vi "AlliGator Convert Gate Image for Export.vi"(8 "error in (no error)":errorcluster, 9 "Exported Gate Image Settings":T1, 10 "Dest Image":T2, 11 "Original Image":T2) -> (0 "error out":errorcluster, 3 "Result Image":T2)   [LabVIEW 2021, in "AlliGator Files.lvlib"]
doc: "Converts a Gate Image (Float) to a U8 or U16 image based on user-selected options."
uses:
  AlliGator Files.lvlib
  <vilib>/vision/Image Controls.llb/IMAQ Image.ctl
  Settings/AlliGator Exported Image Settings.ctl
  <vilib>/Utility/error.llb/Error Cluster From Error Code.vi
  <vilib>/ErrorRing/Error Ring.xnode
  Comparison/Comparison.lvlib
  Settings/AlliGator Settings.lvlib
panel:
  out "dest min value":sgl
  out "dest max value":sgl
  out "source min value":sgl
  out "source max value":sgl
  # "see the AlliGator License on the block diagram (Ctrl+E or Window:Show Block Diagram)"
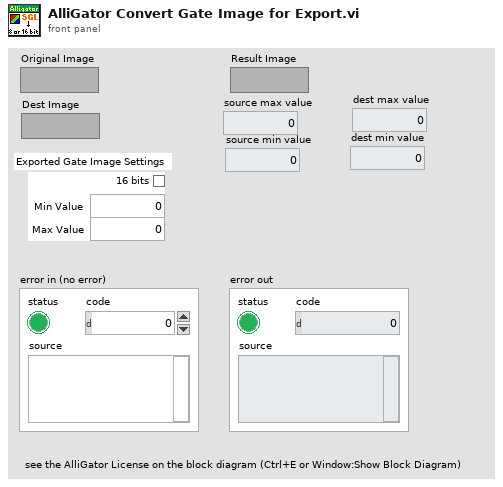
[diagram p1: front panel]
types:
  T1 = typedef "AlliGator Settings.lvlib/AlliGator Exported Image Settings.ctl" = cluster{"bitness":bool, " Min Value":sgl, " Max Value":sgl}
  T2 = typedef "IMAQ Image.ctl" = refnum<image>
  T3 = typedef "Image Type" = u32
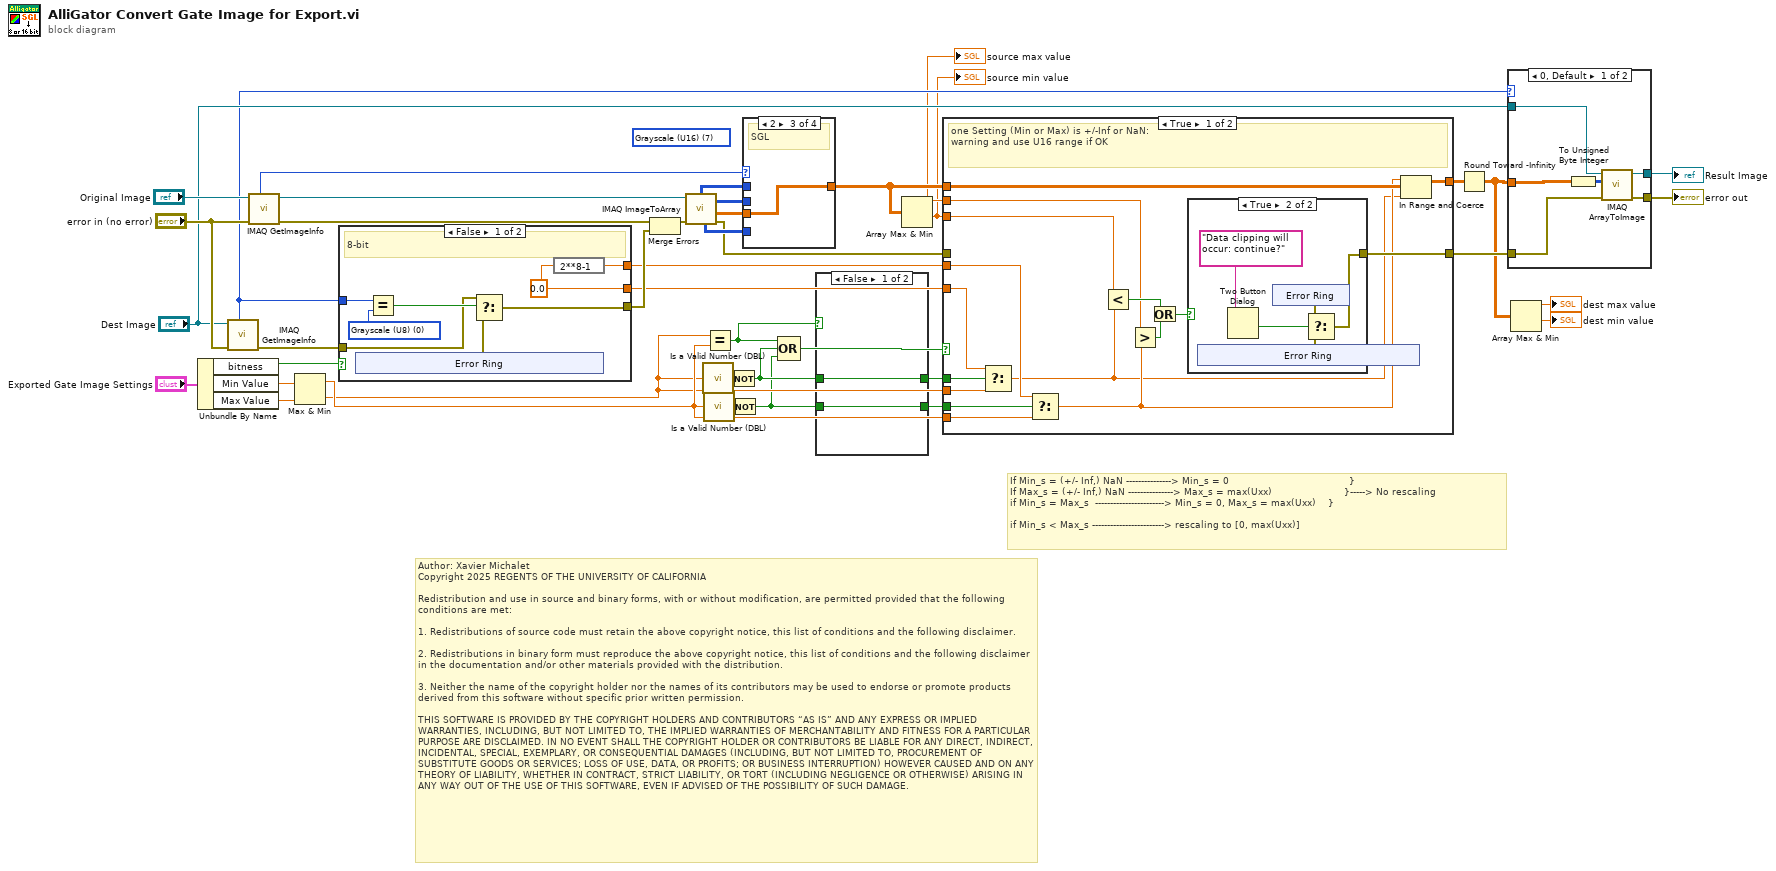
[diagram p0: block diagram]
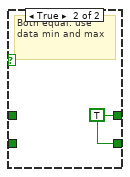
[diagram p2: hidden frame]
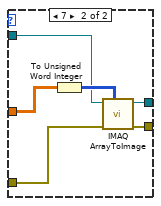
[diagram p3: hidden frame]
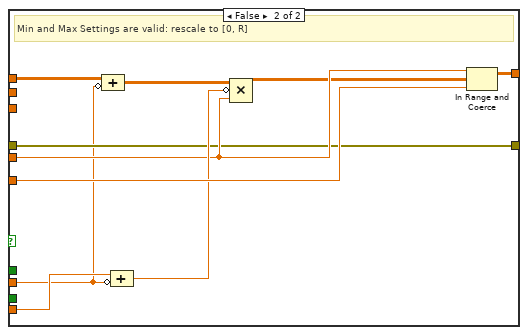
[diagram p5: hidden frame]
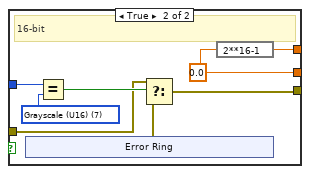
[diagram p6: hidden frame]
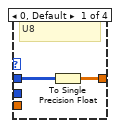
[diagram p7: hidden frame]
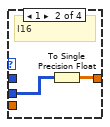
[diagram p8: hidden frame]
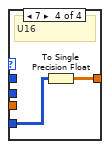
[diagram p9: hidden frame]
diagram:
  (unwired) T3 7 items=["Grayscale (U8)", "Grayscale (I16)", "Grayscale (SGL)", "Complex (CSG)", "RGB (U32)", "HSL (U32)", "RGB (U64)", "Grayscale (U16)"] ("Image Type")
  # "Author: Xavier Michalet\nCopyright 2025 REGENTS OF THE UNIVERSITY OF CALIFORNIA\n\nRedistribution and use in source and binary forms, with or without modification, are permitted provided that the following conditions are met:\n\n1. Redistributions of source code must retain the above copyright notice, this list of conditions and the following disclaimer.\n\n2. Redistributions in binary form must reproduce the above copyright notice, this list of conditions and the following disclaimer in the documentation and/or other materials provided with the distribution.\n\n3. Neither the name of the copyright holder nor the names of its contributors may be used to endorse or promote products derived from this software without specific prior written permission.\n\nTHIS SOFTWARE IS PROVIDED BY THE COPYRIGHT HOLDERS AND CONTRIBUTORS “AS IS” AND ANY EXPRESS OR IMPLIED WARRANTIES, INCLUDING, BUT NOT LIMITED TO, THE IMPLIED WARRANTIES OF MERCHANTABILITY AND FITNESS FOR A PARTICULAR PURPOSE ARE DISCLAIMED. IN NO EVENT SHALL THE COPYRIGHT HOLDER OR CONTRIBUTORS BE LIABLE FOR ANY DIRECT, INDIRECT, INCIDENTAL, SPECIAL, EXEMPLARY, OR CONSEQUENTIAL DAMAGES (INCLUDING, BUT NOT LIMITED TO, PROCUREMENT OF SUBSTITUTE GOODS OR SERVICES; LOSS OF USE, DATA, OR PROFITS; OR BUSINESS INTERRUPTION) HOWEVER CAUSED AND ON ANY THEORY OF LIABILITY, WHETHER IN CONTRACT, STRICT LIABILITY, OR TORT (INCLUDING NEGLIGENCE OR OTHERWISE) ARISING IN ANY WAY OUT OF THE USE OF THIS SOFTWARE, EVEN IF ADVISED OF THE POSSIBILITY OF SUCH DAMAGE."
  # "If Min_s = (+/- Inf,) NaN ---------------> Min_s = 0                                        }\nIf Max_s = (+/- Inf,) NaN ---------------> Max_s = max(Uxx)                        }-----> No rescaling\nif Min_s = Max_s  -----------------------> Min_s = 0, Max_s = max(Uxx)    }\n\nif Min_s < Max_s ------------------------> rescaling to [0, max(Uxx)]"
  n1 = Unbundle By Name("Exported Gate Image Settings") -> ("bitness"=w32:bool, "Min Value"=w9:sgl, "Max Value"=w8:sgl)
  n2 = call "IMAQ GetImageInfo"("error in (no error)"="error in (no error)", "Image"="Dest Image") -> ("error out"=w31:errorcluster, "Image Type"=w19:T3)  [unwired: 2 in, 6 out]
  n3 = call "IMAQ GetImageInfo"("error in (no error)"="error in (no error)", "Image"="Original Image") -> ("error out"=w15:errorcluster, "Image Type"=w39:T3)  [unwired: 2 in, 6 out]
  n4 = Max & Min(x=w9, y=w8) -> (max(x,y)=w5:sgl, min(x,y)=w4:sgl)
  n5 = case shown="False" w32 {
    tunnel: w19 -> [w48 w60]
    tunnel: w31 -> [w45 w57]
    tunnel: [w44 w56] -> w30
    tunnel: [w41 w54] -> w27
    tunnel: [w42 w53] -> w26
    frame False {
      w41 = sgl 0.0 ("Min Value")
      w47 = T3 0 items=["Grayscale (U8)", "Grayscale (I16)", "Grayscale (SGL)", "Complex (CSG)", "RGB (U32)", "HSL (U32)", "RGB (U64)", "Grayscale (U16)"] ("y")
      # "8-bit"
      n6 = xnode "Error Ring"() -> ("error out"=w43:errorcluster)
      n7 = Equal?(x=w48, y=w47) -> (x = y?=w46:bool)
      n8 = Select(t=w45, s=w46, f=w43) -> (s? t:f=w44:errorcluster)
      n9 = expression code="2**8-1"(w41) -> (w42:sgl)
    }
    frame True {
      w54 = sgl 0.0 ("Min Value")
      w59 = T3 7 items=["Grayscale (U8)", "Grayscale (I16)", "Grayscale (SGL)", "Complex (CSG)", "RGB (U32)", "HSL (U32)", "RGB (U64)", "Grayscale (U16)"] ("y")
      # "16-bit"
      n10 = xnode "Error Ring"() -> ("error out"=w55:errorcluster)
      n11 = Equal?(x=w60, y=w59) -> (x = y?=w58:bool)
      n12 = Select(t=w57, s=w58, f=w55) -> (s? t:f=w56:errorcluster)
      n13 = expression code="2**16-1"(w54) -> (w53:sgl)
    }
  }
  n14 = Merge Errors(w15, w30) -> (w16:errorcluster)
  n15 = call "IMAQ ImageToArray"("error in (no error)"=w16, "Image"="Original Image") -> ("Image Pixels (U16)"=w35:u16[][], "Image Pixels (Float)"=w36:sgl[][], "error out"=w18:errorcluster, "Image Pixels (U8)"=w38:u8[][], "Image Pixels (I16)"=w37:i16[][])  [unwired: 2 in]
  n16 = call "Is a Valid Number (DBL).vi"("Number"=w4) -> ("Valid Number?"=w21:bool)  [unwired: 8 in]
  n17 = call "Is a Valid Number (DBL).vi"("Number"=w5) -> ("Valid Number?"=w20:bool)  [unwired: 8 in]
  n18 = Equal?(x=w4, y=w5) -> (x = y?=w7:bool)
  n19 = Not(x=w21) -> (.not. x?=w6:bool)
  n20 = Not(x=w20) -> (.not. x?=w2:bool)
  n21 = case shown="2" w39 {
    tunnel: w38 -> [w66 _ _ _]
    tunnel: w37 -> [_ w68 _ _]
    tunnel: w36 -> [_ _ w69 _]
    tunnel: w35 -> [_ _ _ w71]
    tunnel: [w65 w67 w69 w70] -> w28
    frame 0, Default {
      # "U8"
      n22 = To Single Precision Float(number=w66) -> (single precision float=w65:sgl[][])
    }
    frame 1 {
      # "I16"
      n23 = To Single Precision Float(number=w68) -> (single precision float=w67:sgl[][])
    }
    frame 2 {
      # "SGL"
    }
    frame 7 {
      # "U16"
      n24 = To Single Precision Float(number=w71) -> (single precision float=w70:sgl[][])
    }
  }
  n25 = Compound Arithmetic op=OR(w7, w6, w2) -> (w29:bool)
  n26 = case shown="False" w7 {
    tunnel: w6 -> [w73 _]
    tunnel: [w73 w74] -> w3
    tunnel: w2 -> [w72 _]
    tunnel: [w72 w74] -> w1
    frame False {
    }
    frame True {
      w74 = TRUE
      # "Both equal: use data min and max"
    }
  }
  n27 = Array Max & Min(array=w28) -> (max value=w14:sgl, min value=w13:sgl)  [unwired: 2 out]
  "source max value" <- w14
  "source min value" <- w13
  n28 = case shown="True" w29 {
    tunnel: w28 -> [w87 w110]
    tunnel: w27 -> [w82 w107]
    tunnel: w26 -> [w81 w105]
    tunnel: [w90 w109] -> w25
    tunnel: w5 -> [w80 w102]
    tunnel: w3 -> [w89 _]
    tunnel: w1 -> [w88 _]
    tunnel: w18 -> [_ w104]
    tunnel: [w83 w104] -> w17
    tunnel: w14 -> [w79 _]
    tunnel: w13 -> [w78 _]
    tunnel: w4 -> [w77 w101]
    frame True {
      # "one Setting (Min or Max) is +/-Inf or NaN:\nwarning and use U16 range if OK"
      n29 = Select(t=w82, s=w89, f=w77) -> (s? t:f=w75:sgl)
      n30 = Select(t=w81, s=w88, f=w80) -> (s? t:f=w76:sgl)
      n31 = Less?(x=w78, y=w75) -> (x < y?=w86:bool)
      n32 = Greater?(x=w79, y=w76) -> (0:w85:bool)
      n33 = Or(x=w86, y=w85) -> (x .or. y?=w84:bool)
      n34 = case shown="True" w84 {
        tunnel: [_ w91] -> w83
        frame False {
        }
        frame True {
          n35 = xnode "Error Ring"() -> ("error out"=w92:errorcluster)
          n36 = Two Button Dialog(message="Data clipping will occur: continue?") -> (T button?=w94:bool)  [unwired: 2 in]
          n37 = xnode "Error Ring"() -> ("error out"=w93:errorcluster)
          n38 = Select(t=w93, s=w94, f=w92) -> (s? t:f=w91:errorcluster)
        }
      }
      n39 = In Range and Coerce(upper limit=w76, x=w87, lower limit=w75) -> (coerced(x)=w90:sgl[][])  [unwired: 1 out]
    }
    frame False {
      # "Min and Max Settings are valid: rescale to [0, R]"
      n40 = Compound Arithmetic op=ADD(w110, invert w101) -> (w108:sgl[][])
      n41 = Compound Arithmetic op=ADD(w102, invert w101) -> (w106:sgl)
      n42 = Compound Arithmetic op=MULTIPLY(w108, invert w106, w105) -> (w103:sgl[][])
      n43 = In Range and Coerce(upper limit=w105, x=w103, lower limit=w107) -> (coerced(x)=w109:sgl[][])  [unwired: 1 out]
    }
  }
  n44 = Round Toward -Infinity(1:w25) -> (0:w12:sgl[][])
  n45 = case shown="0, Default" w19 {
    tunnel: [w115 w122] -> w24
    tunnel: [w114 w121] -> w23
    tunnel: w17 -> [w113 w120]
    tunnel: "Dest Image" -> [w112 w118]
    tunnel: w12 -> [w111 w117]
    frame 0, Default {
      n46 = To Unsigned Byte Integer(number=w111) -> (unsigned 8bit integer=w116:u8[][])
      n47 = call "IMAQ ArrayToImage"("error in (no error)"=w113, "Image Pixels (U8)"=w116, "Image"=w112) -> ("error out"=w114:errorcluster, "Image Out"=w115:T2)  [unwired: 7 in]
    }
    frame 7 {
      n48 = To Unsigned Word Integer(number=w117) -> (unsigned 16bit integer=w119:u16[][])
      n49 = call "IMAQ ArrayToImage"("Image Pixels (U16)"=w119, "error in (no error)"=w120, "Image"=w118) -> ("error out"=w121:errorcluster, "Image Out"=w122:T2)  [unwired: 7 in]
    }
  }
  "Result Image" <- w24
  "error out" <- w23
  n50 = Array Max & Min(array=w12) -> (max value=→"dest max value":sgl, min value=→"dest min value":sgl)  [unwired: 2 out]
